vi "NTCP Send Msgs.vi"(0 "Message Type":T2, 1 "Accepted":bool, 2 "NTCP Server In":refnum<k5>, 3 "Combined":bool, 5 "Transaction ID":string, 7 "Contol\nPoint\nSuffix":T1, 9 "ControlPoint name":string, 11 "error in (no error)":errorcluster, 12 "Control Type":bool) -> (6 "Message":string, 13 "NTCP Server Out":refnum<k5>, 15 "error out":errorcluster)   [LabVIEW 2013]
uses:
  Data Access Objects/Metadata/DAO Actions.ctl
  Data Access Objects/Metadata/DAO Actions with Remove.ctl
  Global Data/Transactions/Dataset Source.ctl
  Global Data/Transactions/Dataset Type.ctl
  Apps/Yes No Button.ctl
  Global Data/Transactions/Dataset Transaction Id.ctl
  Control Point Suffix.ctl
  NTCP Msg Types.ctl
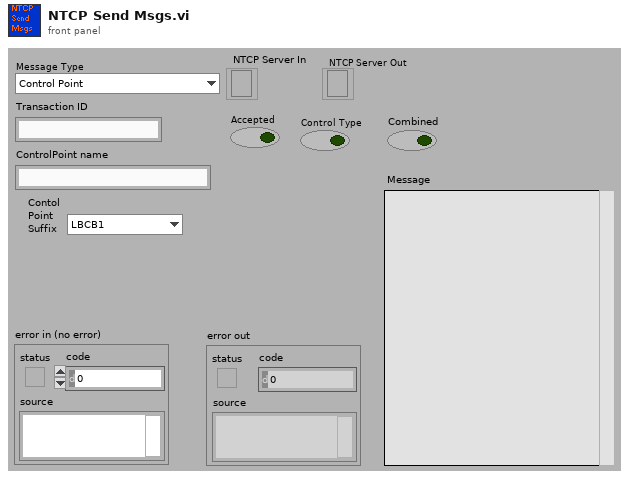
[diagram p1: front panel]
types:
  T1 = typedef "Control Point Suffix.ctl" = enum16{"LBCB1", "LBCB2", "ExternalSensors"}
  T2 = typedef "NTCP Msg Types.ctl" = enum16{"Control Point", "Step Done", "Propose Accepted", "Propose Not Accepted", "Propose Declined", "Propose Response", "Execute Done", "Offsets", "Initial Position"}
  T3 = typedef "Dataset Transaction Id.ctl" = cluster{"Dataset Source":T4, "Dataset Type":T5, "Hold":T6, "Volts":T6, "Tag":string}
  T4 = typedef "Dataset Source.ctl" = enum16{"Continuous", "Hold", "ED", "Volts", "Offsets", "Increments"}
  T5 = typedef "Dataset Type.ctl" = enum16{"LVDT", "Load Cell", "Actuator Command", "Servo Error", "Displacement Command", "Displacement", "Force"}
  T6 = typedef "Yes No Button.ctl" = bool
  T7 = typedef "DAO Actions.ctl" = enum16{"Init", "Get", "Set"}
  T8 = typedef "DAO Actions with Remove.ctl" = enum16{"Init", "Get", "Set", "Remove"}
  T9 = typedef "GlobalOrLocal.ctl" = bool
  T10 = typedef "Source Group Type.ctl" = enum16{"LBCB1", "LBCB2", "Consolidated", "External"}
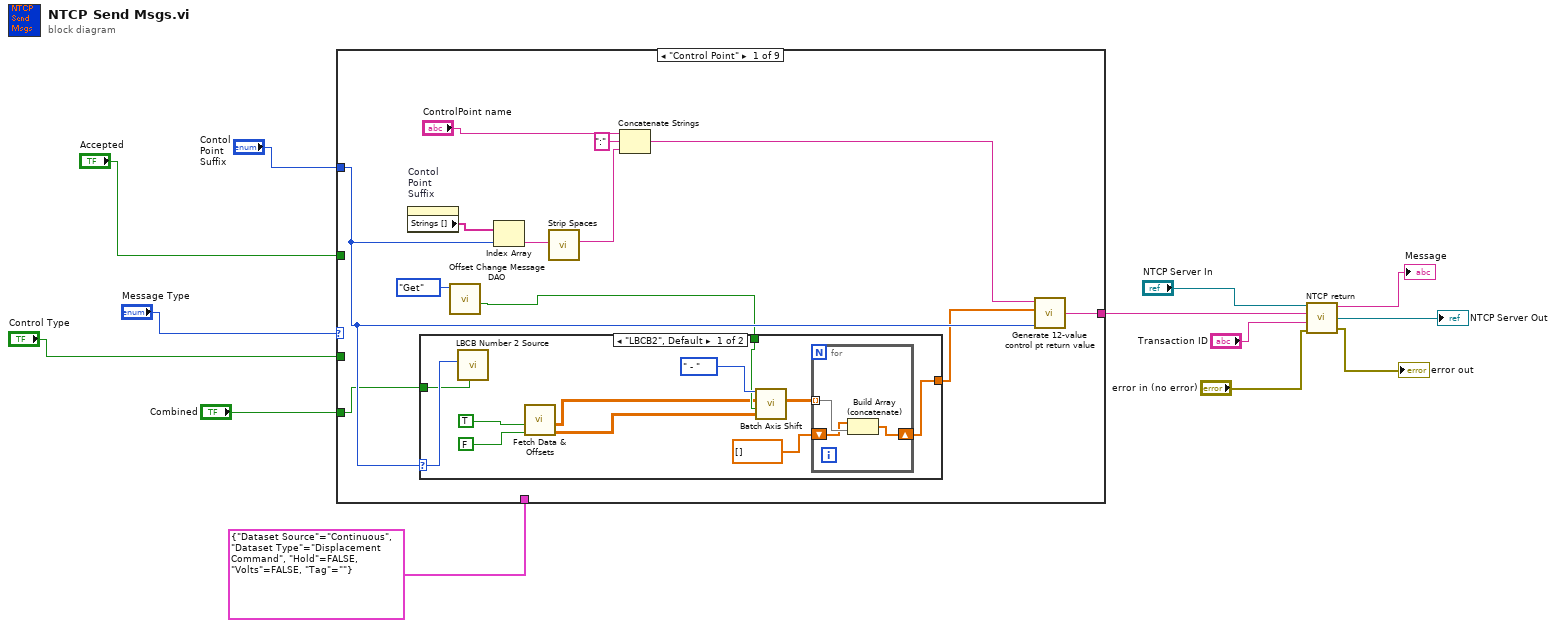
[diagram p0: block diagram]
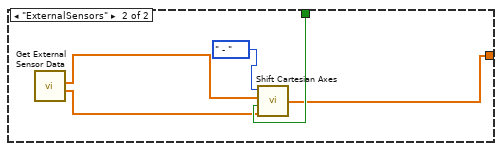
[diagram p2: hidden frame]
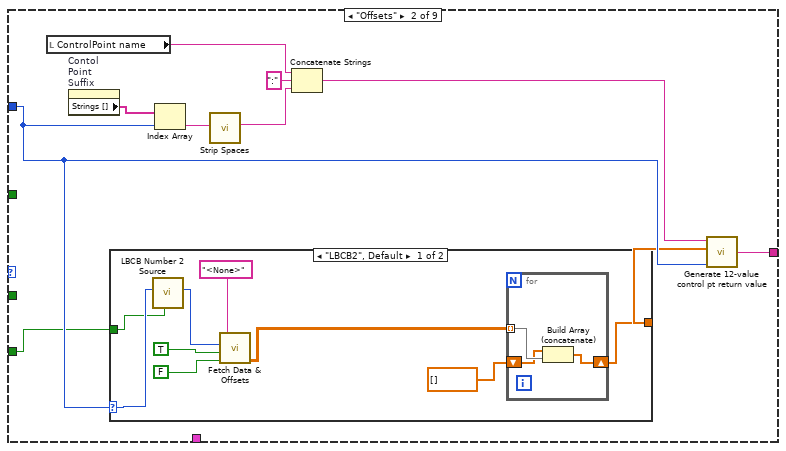
[diagram p3: hidden frame]
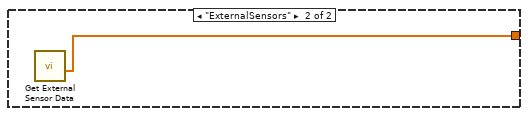
[diagram p4: hidden frame]
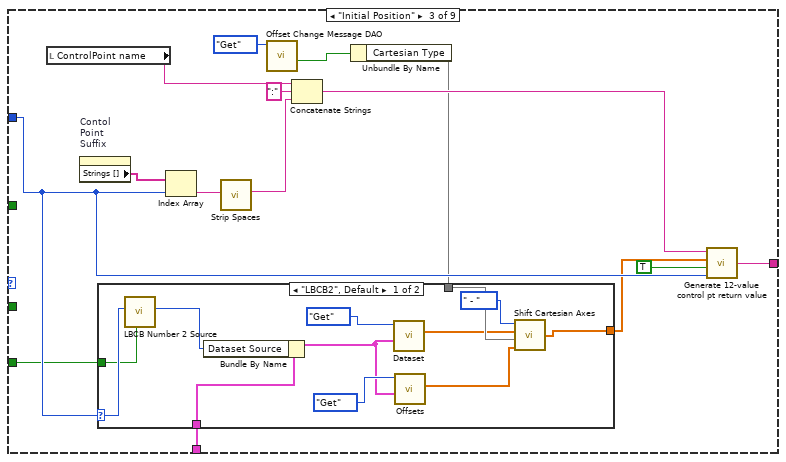
[diagram p5: hidden frame]
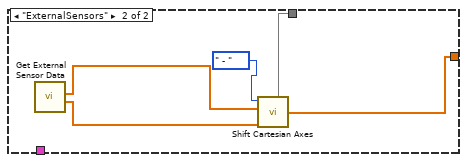
[diagram p6: hidden frame]
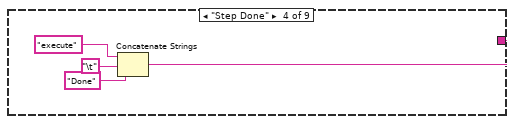
[diagram p7: hidden frame]
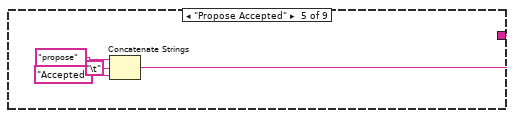
[diagram p8: hidden frame]
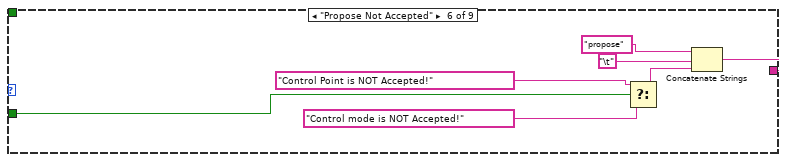
[diagram p9: hidden frame]
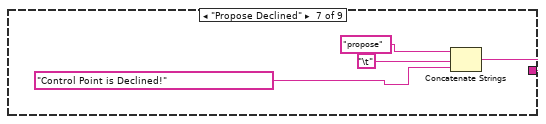
[diagram p10: hidden frame]
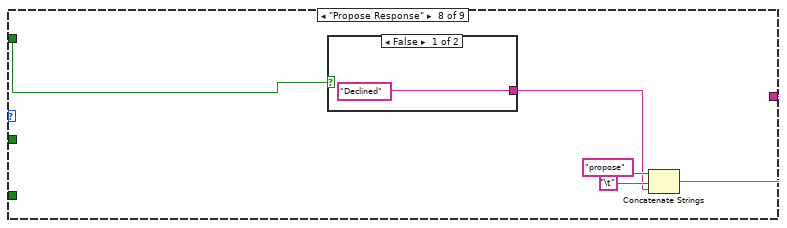
[diagram p11: hidden frame]
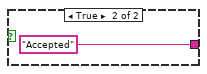
[diagram p12: hidden frame]
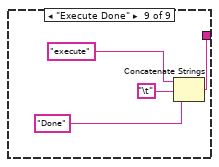
[diagram p13: hidden frame]
diagram:
  n1 = case shown="\"Control Point\"" "Message Type" {
    tunnel: "Control Type" -> [_ _ _ _ _ w110 _ _ _]
    tunnel: "Accepted" -> [_ _ _ _ _ _ _ w121 _]
    tunnel: [w17 w49 w75 w101 w105 w109 w117 w120 w127] -> w9
    tunnel: "Contol\nPoint\nSuffix" -> [w19 w48 w78 _ _ _ _ _ _]
    tunnel: T3 {"Dataset Source"=enum."Continuous", "Dataset Type"=enum."Displacement Command", "Hold"=FALSE, "Volts"=FALSE, "Tag"=""} ("Dataset Trans Id") -> [_ _ w71 _ _ _ _ _ _]
    tunnel: "Combined" -> [w16 w46 w70 _ _ _ _ _ _]
    frame "Control Point" {
      n2 = property on="Contol\nPoint\nSuffix" class="Enum (strict)"() -> ("Strings []"=w23:string[])  [unwired: 2 in, 2 out]
      n3 = call "Offset Change Message DAO.vi"("DAO Actions"=DAO_Actions."Get") -> ("Offset Out"=w14:T9)  [unwired: 8 in, 2 out]
      n4 = case shown="\"LBCB2\", Default" w19 {
        selector: w19 -> [w33 _]
        tunnel: [w34 w43] -> w18
        tunnel: w14 -> [w36 w44]
        tunnel: w16 -> [w31 _]
        frame "LBCB2", Default {
          n5 = call "LBCB Number 2 Source.vi"("Combined"=w31, "LBCB Number"=w33) -> ("Source Group"=w30:T10)  [unwired: 9 in]
          n6 = call "Fetch Data & Offsets.vi"("Include Command"=FALSE, "Include Reading"=TRUE) -> ("Cartesian Offsets"=w28:dbl[][], "Cartesian Data"=w29:dbl[][])  [unwired: 2 in, 2 out]
          n7 = call "Batch Axis Shift.vi"("Offsets In"=w28, "Coordinate Switch"=w36, "Data In"=w29, "Direction"=enum16{" +", " - "}." - ") -> ("Data Out"=w35:dbl[][])  [unwired: 7 in]
          n8 = for {
            shift-right: [w38] -> w34
            shift-left: dbl[] [] -> [w39]
            tunnel: w35 -> [w40] mode=indexing
            n9 = Build Array (concatenate)(w39, w40) -> (w38:dbl[])
          }
        }
        frame "ExternalSensors" {
          n10 = call "Get External Sensor Data.vi"() -> ("Offsets"=w41:dbl[], "Data Out"=w42:dbl[])  [unwired: 8 in, 2 out]
          n11 = call "Shift Cartesian Axes.vi"("Coordinate Offset"=w41, "Coordinate Switch"=w44, "Coordinate Input"=w42, "Direction"=enum16{" +", " - "}." - ") -> ("Coordinate Output"=w43:dbl[])
        }
      }
      n12 = Index Array(array=w23, index=w19) -> (element=w21:string)
      n13 = call "Strip Spaces.vi"("input string"=w21) -> ("result string"=w20:string)  [unwired: 10 out]
      n14 = Concatenate Strings("ControlPoint name", ":" ("string"), w20) -> (w22:string)
      n15 = call "Generate 12-value control pt return value.vi"("Contol\nPoint\nSuffix"=w19, "Hold Data"=w18, "ControlPoint name"=w22) -> ("concatenated string"=w17:string)  [unwired: 1 in]
    }
    frame "Offsets" {
      n16 = local read "ControlPoint name"() -> (w50:string)
      n17 = property on="Contol\nPoint\nSuffix" class="Enum (strict)"() -> ("Strings []"=w54:string[])  [unwired: 2 in, 2 out]
      n18 = case shown="\"LBCB2\", Default" w48 {
        selector: w48 -> [w60 _]
        tunnel: [w56 w68] -> w47
        tunnel: w46 -> [w59 _]
        frame "LBCB2", Default {
          n19 = call "LBCB Number 2 Source.vi"("Combined"=w59, "LBCB Number"=w60) -> ("Source Group"=w63:T10)  [unwired: 9 in]
          n20 = call "Fetch Data & Offsets.vi"("Include Command"=FALSE, "Include Reading"=TRUE, "Source"=w63, "Dataset Source"="<None>" ("Force Tag")) -> ("Cartesian Offsets"=w57:dbl[][])  [unwired: 3 out]
          n21 = for {
            shift-right: [w65] -> w56
            shift-left: dbl[] [] -> [w66]
            tunnel: w57 -> [w67] mode=indexing
            n22 = Build Array (concatenate)(w66, w67) -> (w65:dbl[])
          }
        }
        frame "ExternalSensors" {
          n23 = call "Get External Sensor Data.vi"() -> ("Offsets"=w68:dbl[])  [unwired: 8 in, 3 out]
        }
      }
      n24 = Index Array(array=w54, index=w48) -> (element=w52:string)
      n25 = call "Strip Spaces.vi"("input string"=w52) -> ("result string"=w51:string)  [unwired: 10 out]
      n26 = Concatenate Strings(w50, ":" ("string"), w51) -> (w53:string)
      n27 = call "Generate 12-value control pt return value.vi"("Contol\nPoint\nSuffix"=w48, "Hold Data"=w47, "ControlPoint name"=w53) -> ("concatenated string"=w49:string)  [unwired: 1 in]
    }
    frame "Initial Position" {
      n28 = local read "ControlPoint name"() -> (w76:string)
      n29 = property on="Contol\nPoint\nSuffix" class="Enum (strict)"() -> ("Strings []"=w82:string[])  [unwired: 2 in, 2 out]
      n30 = Index Array(array=w82, index=w78) -> (element=w80:string)
      n31 = call "Strip Spaces.vi"("input string"=w80) -> ("result string"=w79:string)  [unwired: 10 out]
      n32 = call "Offset Change Message DAO.vi"("DAO Actions"=DAO_Actions."Get") -> ("Offset Out"=w73:T9)  [unwired: 8 in, 2 out]
      n33 = Concatenate Strings(w76, ":" ("string"), w79) -> (w81:string)
      n34 = Unbundle By Name(w73) -> ("Cartesian Type"=w72)
      n35 = case shown="\"LBCB2\", Default" w78 {
        selector: w78 -> [w95 _]
        tunnel: [w89 w96] -> w77
        tunnel: w72 -> [w88 w97]
        tunnel: w71 -> [w92 _]
        tunnel: w70 -> [w84 _]
        frame "LBCB2", Default {
          n36 = call "LBCB Number 2 Source.vi"("Combined"=w84, "LBCB Number"=w95) -> ("Source Group"=w90:T10)  [unwired: 9 in]
          n37 = Bundle By Name(cluster=w92, "Dataset Source"=w90) -> (w91:T3)
          n38 = call "Dataset.vi"("Group ID"=w91, "DAO Actions"=DAO_Actions."Get") -> ("Data Out"=w86:dbl[])  [unwired: 7 in, 2 out]
          n39 = call "Offsets.vi"("Dataset Trans Id"=w91, "DAO Actions"=DAO_Actions_with_Remove."Get") -> ("Data Out"=w85:dbl[])  [unwired: 7 in, 2 out]
          n40 = call "Shift Cartesian Axes.vi"("Coordinate Offset"=w85, "Coordinate Switch"=w88, "Coordinate Input"=w86, "Direction"=enum16{" +", " - "}." - ") -> ("Coordinate Output"=w89:dbl[])
        }
        frame "ExternalSensors" {
          n41 = call "Get External Sensor Data.vi"() -> ("Offsets"=w98:dbl[], "Data Out"=w99:dbl[])  [unwired: 8 in, 2 out]
          n42 = call "Shift Cartesian Axes.vi"("Coordinate Offset"=w98, "Coordinate Switch"=w97, "Coordinate Input"=w99, "Direction"=enum16{" +", " - "}." - ") -> ("Coordinate Output"=w96:dbl[])
        }
      }
      n43 = call "Generate 12-value control pt return value.vi"("Contol\nPoint\nSuffix"=w78, "Displacements Only"=TRUE, "Hold Data"=w77, "ControlPoint name"=w81) -> ("concatenated string"=w75:string)
    }
    frame "Step Done" {
      n44 = Concatenate Strings("execute", "\t", "Done") -> (w101:string)
    }
    frame "Propose Accepted" {
      n45 = Concatenate Strings("propose", "\t", "Accepted") -> (w105:string)
    }
    frame "Propose Not Accepted" {
      n46 = Select(t="Control Point is NOT Accepted!", s=w110, f="Control mode is NOT Accepted!") -> (s? t:f=w113:string)
      n47 = Concatenate Strings("propose", "\t", w113) -> (w109:string)
    }
    frame "Propose Declined" {
      n48 = Concatenate Strings("propose", "\t", "Control Point is Declined!") -> (w117:string)
    }
    frame "Propose Response" {
      n49 = case shown="False" w121 {
        tunnel: ["Declined" "Accepted"] -> w122
        frame False {
        }
        frame True {
        }
      }
      n50 = Concatenate Strings("propose", "\t", w122) -> (w120:string)
    }
    frame "Execute Done" {
      n51 = Concatenate Strings("execute", "\t", "Done") -> (w127:string)
    }
  }
  n52 = call "NTCP return.vi"("NTCP Server"="NTCP Server In", "Message Body"=w9, "Transaction ID"="Transaction ID", "NTCP return error"="error in (no error)") -> ("Response string"=→"Message":string, "connection ID out"=→"NTCP Server Out":refnum<k5>, "error out"=→"error out":errorcluster)  [unwired: 1 in]
